vi "DT3120_AquireFrame.vi"(8 "error in (no error)":errorcluster, 9 "Image":T1, 10 "Frame Size":T2, 11 "DevId":i32) -> (0 "error out":errorcluster, 1 "Image Out":T1, 2 "Frame":u8[][](array[numeric]), 3 "DevId (dup)":i32)   [LabVIEW 2010]
uses:
  <vilib>/vision/Image Controls.llb/IMAQ Image.ctl
  Libs/olfg32.dll
panel:
  out "BufSize":u32
  out "FrameId":u32
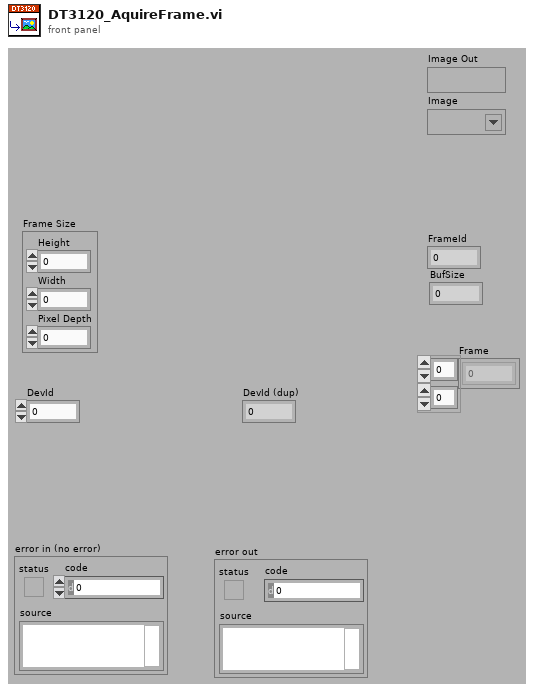
[diagram p1: front panel]
types:
  T1 = typedef "IMAQ Image.ctl" = refnum<image>
  T2 = cluster{"Height":u32, "Width":u32, "Pixel Depth":u32}
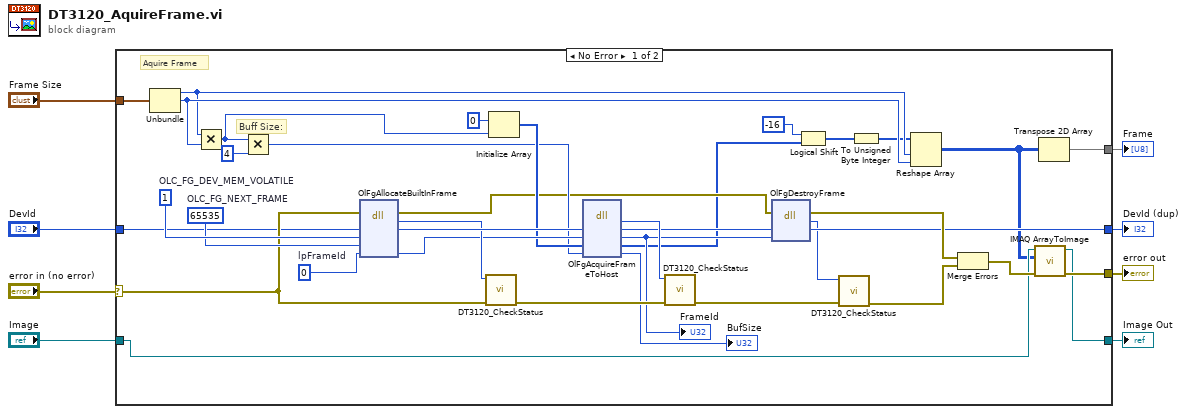
[diagram p0: block diagram]
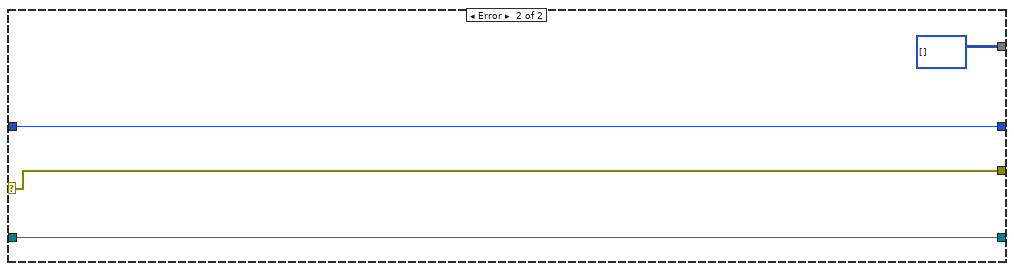
[diagram p2: hidden frame]
diagram:
  n1 = case shown="No Error" "error in (no error)" {
    selector: "error in (no error)" -> [w37 w49]
    tunnel: "DevId" -> [w36 w48]
    tunnel: [w15 w49] -> w7
    tunnel: [w24 w48] -> w6
    tunnel: "Frame Size" -> [w43 _]
    tunnel: [w9 u8[][] [] ("lpBuffer")] -> w3
    tunnel: [w14 w46] -> w2
    tunnel: "Image" -> [w13 w46]
    frame No Error {
      w38 = u32 0  # lpFrameId
      w39 = u16 65535  # OLC_FG_NEXT_FRAME
      w40 = 1  # OLC_FG_DEV_MEM_VOLATILE
      # "Buff Size:"
      # "Aquire Frame"
      n2 = Unbundle(w43) -> ("Height"=w30:u32, "Width"=w31:u32)  [unwired: 1 out]
      n3 = Multiply(x=w30, y=w31) -> (x*y=w27:u32)
      n4 = Multiply(x=w27, y=u32 4) -> (x*y=w28:u32)
      n5 = dll-call lib="C:/LabVIEW Programs/newMicroTime/Libs/olfg32.dll" fn="OlFgAllocateBuiltInFrame"(error in=w37, "DevId"=w36, "MemType"=w40, "BufNum"=w39, "lpFrameId"=w38) -> (error out=w19:errorcluster, "Status"=w34:u32, "DevId"=w35:i32, "lpFrameId"=w33:u32)  [unwired: 4 in, 1 out]
      n6 = call "DT3120_CheckStatus.vi"("error in"=w37, "Status"=w34) -> ("error out"=w45:errorcluster)  [unwired: 9 out]
      n7 = Initialize Array(u32 0 ("element"), w27) -> (w32:u32[])
      n8 = dll-call lib="C:/LabVIEW Programs/newMicroTime/Libs/olfg32.dll" fn="OlFgAcquireFrameToHost"("DevId"=w35, "FrameId"=w33, "lpBuffer"=w32, "BufSize"=w28) -> ("Status"=w44:u32, "DevId"=w25:i32, "FrameId"=w23:u32, "lpBuffer"=w18:u32[], "BufSize"=→"BufSize":u32)  [unwired: 3 in, 2 out]
      "FrameId" <- w23
      n9 = call "DT3120_CheckStatus.vi"("error in"=w45, "Status"=w44) -> ("error out"=w21:errorcluster)  [unwired: 9 out]
      n10 = dll-call lib="C:/LabVIEW Programs/newMicroTime/Libs/olfg32.dll" fn="OlFgDestroyFrame"(error in=w19, "DevId"=w25, "FrameId"=w23) -> (error out=w26:errorcluster, "Status"=w22:u32, "DevId"=w24:i32)  [unwired: 3 in, 1 out]
      n11 = Logical Shift(y=i8 -16, x=w18) -> (x << y=w12:u32[])
      n12 = call "DT3120_CheckStatus.vi"("error in"=w21, "Status"=w22) -> ("error out"=w20:errorcluster)  [unwired: 9 out]
      n13 = To Unsigned Byte Integer(number=w12) -> (unsigned 8bit integer=w11:u8[])
      n14 = Reshape Array(w11, w30, w31) -> (w10:u8[][])
      n15 = Merge Errors(w26, w20) -> (w16:errorcluster)
      n16 = call "IMAQ ArrayToImage"("error in (no error)"=w16, "Image Pixels (U8)"=w10, "Image"=w13) -> ("error out"=w15:errorcluster, "Image Out"=w14:T1)  [unwired: 7 in]
      n17 = Transpose 2D Array(2D array=w10) -> (transposed array=w9:u8[][])
    }
    frame Error {
    }
  }
  "error out" <- w7
  "DevId (dup)" <- w6
  "Frame" <- w3
  "Image Out" <- w2
